vi "Multi-output Decision Tree Regression.vi"() -> ()   [LabVIEW 2020]
doc: "An example to illustrate multi-output regression with decision tree.\n\nThe decision trees is used to predict simultaneously the noisy x and y observations of a circle given a single underlying feature. As a result, it learns local linear regressions approximating the circle.\n\nWe can see that if the maximum depth of the tree (controlled by the max_depth parameter) is set too high, the decision trees learn too fine details of the training data and learn from the noise, i.e. they overfit."
uses:
  Model/Supervised/Tree/DecisionTreeRegressor/Controls/decision_tree_regressor_params.ctl
  Model/Supervised/Tree/DecisionTreeRegressor/DecisionTreeRegressor.lvclass
  C:/Users/cipop/TDF Dropbox/2_Technologies de France/1 - Services et Etudes/PLAIY/2 - DEV/PLAIYLAB/code/Model/Model.lvclass
  C:/Users/cipop/TDF Dropbox/2_Technologies de France/1 - Services et Etudes/PLAIY/2 - DEV/PLAIYLAB/code/Model/Supervised/Tree/Tree.lvclass
  Model/Supervised/Tree/DecisionTreeRegressor/DecisionTreeRegressor.vi
panel:
  in  "error in":errorcluster
  in  "X_test":dbl[][](array[numeric])=array20000x1[20000 elements]
  in  "Y":dbl[][](array[numeric])=[[1.8256976133184155, 2.6449015931558], [2.8069433208733265, 1.4109123270047574], [-2.720432252800947, -1.5712583361782755], [-2.993723955966916, -0.9524816410614725], [-0.852188059374447, 3.0238022277505143], [2.3890282910556984, -1.3300710818645851], [-2.7953490289874754, -1.4337462143727313], [-3.0739434689186576, 0.6484411700236866], [-3.035155908655832, 0.8108224289207518], [0.4667646891222363, 3.106724179272756], [2.657323005508145, 0.5622915200653608], [2.6321235585609952, -1.7150889112689056], [2.2861793518787192, -2.1547594696700503], [-3.131091686155956, -0.25665006131775714], [3.09796044300452, 0.52177149660421], [1.2566356253877626, -3.4745833366109107], [-0.3508125342066263, -3.1219441005458255], [-1.029946994677885, -2.967964553232291], [-3.1400292397187446, 0.09909982240488503], [-3.139440982914441, 0.11625281023083907], [2.374924854338179, -2.310100563289901], [0.1898574871704973, -3.135850528270546], [0.26325593502023165, 3.1305431978757268], [1.998387653083125, -2.424056762762431], [-1.7235342528252657, -2.6266012412293214], [-2.507857486775842, 1.715435086269062], [-2.2807611493251936, -2.1604936891410214], [-0.7260634523667222, -3.0565399170020133], [-2.813177057014104, -1.3984417209804716], [0.22316518691925616, 3.1336562830720043], [2.7072417339618564, -0.09180969787531168], [1.328074566794052, -2.8470725923523883], [-3.0330950538704733, -0.8184978895976633], [1.1767886156655354, 2.9128633601886222], [2.258533538271828, 2.1837194548729686], [2.0169505446781475, 2.4581823603746082], [2.5898528068960425, 1.778276367638632], [2.9230441084338596, 1.1512677973605707], [-3.061595888228995, -0.704439506465011], [-3.138513218222494, -0.13906538078199607], [1.1882465114137004, 2.3680122824827508], [3.128889883239954, -0.2822277442917763], [3.1209808517306605, -0.35928112143545593], [2.4365611927984574, -1.9831222743033061], [2.320560298326097, -2.117688433864163], [1.163818201165327, -2.4488127202110106], [0.22133561986844763, -3.1337860399948823], [-3.0480845941241945, -0.7607790140061058], [2.6376306285752116, -1.7066074734077816], [1.7551500436024252, -2.6055810725309936], [-2.640875958769442, 0.11463798380303492], [0.5122025995369903, -3.099556887381954], [1.0768665573344194, 2.9512646134808165], [2.4532511789429097, 1.96243803828416], [3.1286979062077664, 0.2843480486665858], [-1.8432014614152683, 2.377668793227683], [2.595118339887417, -1.7705832945866549], [2.430215435157508, -1.9908936033378486], [0.09436047647264918, -3.1401752342137232], [-3.1399592202002538, 0.10129410925011163], [-2.9838035181445264, 1.6890017291269777], [-3.1138635263815986, -0.4164833011775086], [-2.2395802491581875, 2.20315335568587], [-1.2184723923859657, 2.8956742617363886], [3.002738180455847, 0.923670840030184], [3.0076138641555845, 0.3674314765799399], [1.4060012437714013, -2.8094065038015823], [-2.9388665139979615, -1.1102558326758865], [-1.9142577560461527, 2.4910282303712465], [-1.2202862616970438, 2.894910333775955], [2.3422131280375744, 2.6709038209071414], [2.1766010669755884, 2.265394490222418], [2.9058348451257574, 1.1940386316791947], [2.4393286440630204, -1.9797171937787035], [0.25920539036144385, 3.13088118054597], [2.8615826236106736, 0.6179612178483794], [-1.8568171941699843, 2.5341338379264946], [-0.7364447224204342, 3.054055266675514], [-0.3232054114594505, 3.124922825141876], [-0.24165004579056773, 3.1322850535126547], [2.972047565800148, 1.299914590322177], [-1.3909118919367747, -2.8169076147360994], [-3.0677792098733216, 0.6770045203382145], [-2.5585023948376673, -1.8230934964228462], [-0.37731343682908297, 3.1188521881419105], [0.4010838370305029, 3.32924687119214], [0.717059789905144, 3.0586646855761335], [2.9939436325287945, 0.9517909047315192], [-1.1697036424392835, -2.915715656567634], [-1.8696557692167248, -2.524676554674673], [-2.959968196291449, 1.7949709876659181], [-2.64529910590806, 1.6946967402374318], [0.1183836979789325, 3.1393613524317634], [-1.972269507042122, -2.4453542468691896], [2.5633577388920226, 1.8162603072114238], [2.5739321091870977, -1.3610566109470112], [-1.4275971586239513, -2.7984943726543707], [-3.009488498821716, 0.9014340666677573], [-1.762098393366606, 2.6008870896646368], [-1.173578057741207, -2.914158359368573]]
  in  "X":dbl[][](array[numeric])=[[-99.97712503653102], [-99.4259345937682], [-96.34234453116164], [-96.12660842594059], [-94.52248136041477], [-92.18904335342353], [-90.00930821078256], [-89.32749097658393], [-82.99115772604442], [-81.53228104624044], [-80.33063323338999], [-79.53311423443483], [-79.3547986844716], [-77.05080540932497], [-73.99428557634447], [-72.5050591707525], [-72.14473054984829], [-71.92261228095325], [-70.65428501883797], [-70.64882183657738], [-66.92916057661344], [-66.03391608708623], [-62.74795772446582], [-60.37970218302424], [-59.109550053696516], [-57.674376799988195], [-52.59460395139446], [-46.890668125554754], [-46.01442164699478], [-43.91120158711897], [-42.44493228273025], [-41.2771703252641], [-39.53348547363205], [-37.31516436815143], [-36.89687379878741], [-30.88785459139045], [-30.446828050898688], [-30.220331604431493], [-20.646505153866016], [-20.46463260289329], [-18.372639447743765], [-17.188802436086334], [-17.16414609461947], [-16.595599059485195], [-16.539039526574612], [-16.161097119341036], [-15.778474998989566], [-14.381762025741011], [-10.421294764818967], [-10.01757330401189], [-1.6853681439323367], [2.9778224116617196], [6.6330569946034075], [7.179281183102319], [7.7633468006713855], [11.737965689150329], [14.735897334457178], [14.823521098402608], [15.677922877426354], [17.31100810039858], [17.861107380656847], [23.428982724144774], [24.339144041824355], [24.73444141112178], [32.68829956368961], [32.75892904395775], [34.093502035680444], [35.76710658797819], [37.043900079351886], [37.30018553631675], [38.37542279009466], [38.464523133862826], [38.88003154554903], [39.951672004186236], [44.06489868843161], [45.199597070090306], [49.63313087596788], [50.028862988993495], [50.162420627231114], [50.18848680546745], [57.85586569029769], [60.14891373510733], [61.47825774190477], [66.92513437947457], [75.27783045920765], [75.62348727818909], [75.62850068588261], [76.66121824116198], [78.92133270076945], [79.17724363921337], [80.67590411245075], [80.6803830575767], [81.71910061861911], [85.50171607920677], [88.91895119816266], [89.89785174141426], [91.5779060301004], [92.96800942967712], [93.65231514387949], [97.77221778129893]]
  out "error out":errorcluster caption="sortie d'erreur"
  out "XY Graph":cluster{"X":dbl[], "Y":dbl[]}[](graph) caption="Multi-outpout Decision Tree Regression"
  out "y_3":dbl[][](array[numeric])
  out "y_2":dbl[][](array[numeric])
  out "y_1":dbl[][](array[numeric])
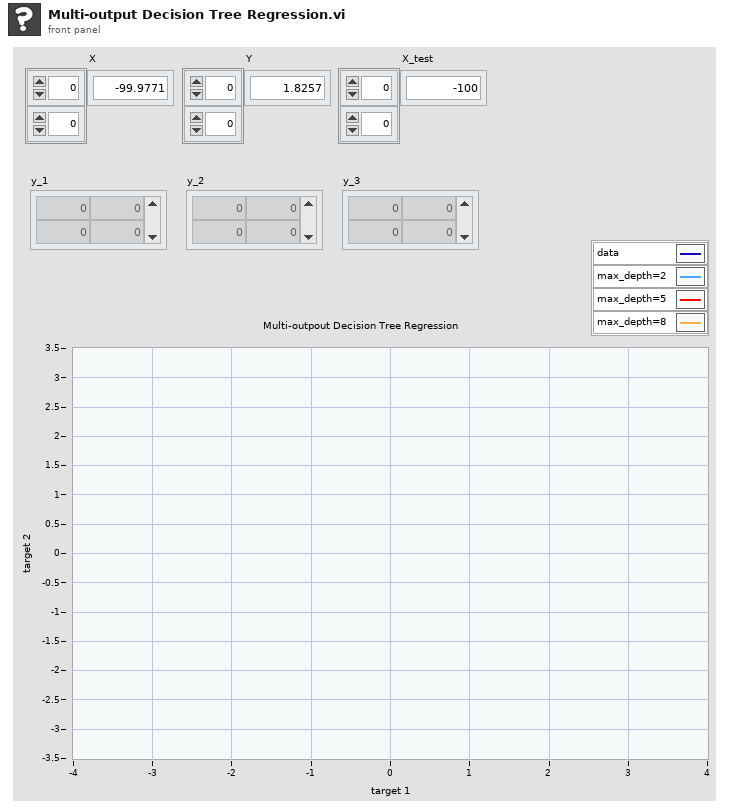
[diagram p1: front panel]
types:
  T1 = cluster{"max_depth_type":string, "max_depth_int":dbl}
  T2 = typedef "decision_tree_regressor_params.ctl" = cluster{"criterion":string, "splitter":string, "max_depth":cluster{"max_depth_type":string, "max_depth_int":dbl}, "min_samples_split":dbl, "min_samples_leaf":dbl, "min_weight_fraction_leaf":dbl, "max_features":cluster{"max_features_type":string, "max_features_int":dbl, "max_features_float":dbl}, "random_state":dbl, "max_leaf_nodes":cluster{"max_leaf_nodes_type":string, "max_leaf_nodes_int":dbl}, "min_impurity_decrease":dbl, "ccp_alpha":dbl}
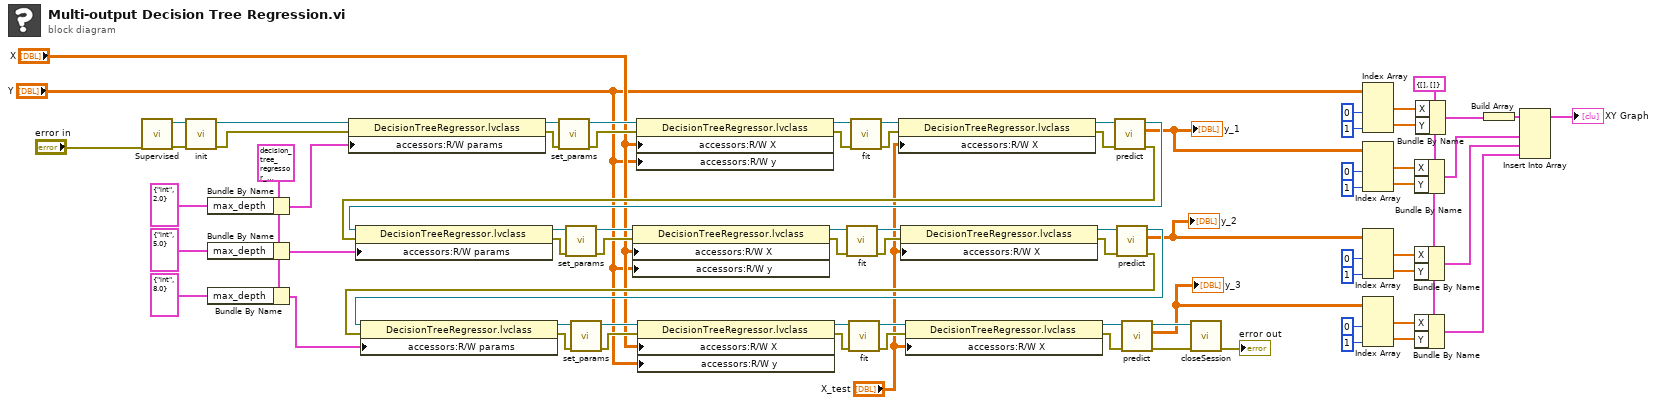
[diagram p0: block diagram]
diagram:
  w7 = cluster{"X":dbl[], "Y":dbl[]} {"X"=[], "Y"=[]}
  w44 = T2 {"criterion"="mse", "splitter"="best", "max_depth"={"max_depth_type"="None", "max_depth_int"=0.0}, "min_samples_split"=2.0, "min_samples_leaf"=1.0, "min_weight_fraction_leaf"=0.0, "max_features"={"max_features_type"="None", "max_features_int"=0.0, "max_features_float"=0.0}, "random_state"=0.0, "max_leaf_nodes"={"max_leaf_nodes_type"="None", "max_leaf_nodes_int"=0.0}, "min_impurity_decrease"=0.0, "ccp_alpha"=0.0} ("R/W params")
  n1 = call-poly "Supervised.vi"("error in"="error in") -> ("error out"=w76:errorcluster, "out"=w77:refnum<class "DecisionTreeRegressor.lvclass">)  [unwired: 9 in]
  n2 = call-dynamic "init.vi"("error in (no error)"=w76, "Model en entrée"=w77) -> ("error out"=w74:errorcluster, "Model en sortie"=w75:refnum<class "DecisionTreeRegressor.lvclass">)  [unwired: 8 in]
  n3 = Bundle By Name(cluster=w44, "max_depth"=T1 {"max_depth_type"="int", "max_depth_int"=2.0}) -> (w49:T2)
  n4 = Bundle By Name(cluster=w44, "max_depth"=T1 {"max_depth_type"="int", "max_depth_int"=5.0}) -> (w47:T2)
  n5 = Bundle By Name(cluster=w44, "max_depth"=T1 {"max_depth_type"="int", "max_depth_int"=8.0}) -> (w45:T2)
  n6 = property class="DecisionTreeRegressor.lvclass"(reference=w75, error in=w74, "accessors:R/W params"=w49) -> (reference out=w73:refnum<class "DecisionTreeRegressor.lvclass">, error out=w72:errorcluster)
  n7 = call-dynamic "set_params.vi"("error in (no error)"=w72, "DecisionTreeRegressor.lvclass 2"=w73) -> ("error out"=w78:errorcluster, "DecisionTreeRegressor.lvclass"=w71:refnum<class "DecisionTreeRegressor.lvclass">)  [unwired: 8 in]
  n8 = property class="DecisionTreeRegressor.lvclass"(reference=w71, error in=w78, "accessors:R/W X"="X", "accessors:R/W y"="Y") -> (reference out=w70:refnum<class "DecisionTreeRegressor.lvclass">, error out=w69:errorcluster)
  n9 = call-dynamic "fit.vi"("error in (no error)"=w69, "Tree.lvclass 2"=w70) -> ("error out"=w5:errorcluster, "Tree.lvclass"=w68:refnum<class "DecisionTreeRegressor.lvclass">)  [unwired: 8 in]
  n10 = property class="DecisionTreeRegressor.lvclass"(reference=w68, error in=w5, "accessors:R/W X"="X_test") -> (reference out=w67:refnum<class "DecisionTreeRegressor.lvclass">, error out=w66:errorcluster)
  n11 = call-dynamic "predict.vi"("error in (no error)"=w66, "Tree.lvclass 2"=w67) -> ("error out"=w43:errorcluster, "C"=w24:dbl[][], "Tree.lvclass"=w42:refnum<class "DecisionTreeRegressor.lvclass">)  [unwired: 7 in]
  "y_1" <- w24
  n12 = property class="DecisionTreeRegressor.lvclass"(reference=w42, error in=w43, "accessors:R/W params"=w47) -> (reference out=w62:refnum<class "DecisionTreeRegressor.lvclass">, error out=w63:errorcluster)
  n13 = call-dynamic "set_params.vi"("error in (no error)"=w63, "DecisionTreeRegressor.lvclass 2"=w62) -> ("error out"=w39:errorcluster, "DecisionTreeRegressor.lvclass"=w61:refnum<class "DecisionTreeRegressor.lvclass">)  [unwired: 8 in]
  n14 = property class="DecisionTreeRegressor.lvclass"(reference=w61, error in=w39, "accessors:R/W X"="X", "accessors:R/W y"="Y") -> (reference out=w40:refnum<class "DecisionTreeRegressor.lvclass">, error out=w64:errorcluster)
  n15 = call-dynamic "fit.vi"("error in (no error)"=w64, "Tree.lvclass 2"=w40) -> ("error out"=w37:errorcluster, "Tree.lvclass"=w38:refnum<class "DecisionTreeRegressor.lvclass">)  [unwired: 8 in]
  n16 = property class="DecisionTreeRegressor.lvclass"(reference=w38, error in=w37, "accessors:R/W X"="X_test") -> (reference out=w36:refnum<class "DecisionTreeRegressor.lvclass">, error out=w65:errorcluster)
  n17 = call-dynamic "predict.vi"("error in (no error)"=w65, "Tree.lvclass 2"=w36) -> ("error out"=w41:errorcluster, "C"=w14:dbl[][], "Tree.lvclass"=w35:refnum<class "DecisionTreeRegressor.lvclass">)  [unwired: 7 in]
  "y_2" <- w14
  n18 = property class="DecisionTreeRegressor.lvclass"(reference=w35, error in=w41, "accessors:R/W params"=w45) -> (reference out=w52:refnum<class "DecisionTreeRegressor.lvclass">, error out=w53:errorcluster)
  n19 = call-dynamic "set_params.vi"("error in (no error)"=w53, "DecisionTreeRegressor.lvclass 2"=w52) -> ("error out"=w51:errorcluster, "DecisionTreeRegressor.lvclass"=w54:refnum<class "DecisionTreeRegressor.lvclass">)  [unwired: 8 in]
  n20 = property class="DecisionTreeRegressor.lvclass"(reference=w54, error in=w51, "accessors:R/W X"="X", "accessors:R/W y"="Y") -> (reference out=w55:refnum<class "DecisionTreeRegressor.lvclass">, error out=w56:errorcluster)
  n21 = call-dynamic "fit.vi"("error in (no error)"=w56, "Tree.lvclass 2"=w55) -> ("error out"=w58:errorcluster, "Tree.lvclass"=w57:refnum<class "DecisionTreeRegressor.lvclass">)  [unwired: 8 in]
  n22 = property class="DecisionTreeRegressor.lvclass"(reference=w57, error in=w58, "accessors:R/W X"="X_test") -> (reference out=w59:refnum<class "DecisionTreeRegressor.lvclass">, error out=w60:errorcluster)
  n23 = call-dynamic "predict.vi"("error in (no error)"=w60, "Tree.lvclass 2"=w59) -> ("error out"=w33:errorcluster, "C"=w9:dbl[][], "Tree.lvclass"=w34:refnum<class "DecisionTreeRegressor.lvclass">)  [unwired: 7 in]
  "y_3" <- w9
  n24 = call-dynamic "closeSession.vi"("error in"=w33, "Python en entrée"=w34) -> ("error out"=→"error out":errorcluster)  [unwired: 8 in, 1 out]
  n25 = Index Array(array="Y", index (col) #1=0 ("disabled index (col)"), index (col) #2=1 ("index (col)")) -> (element #1=w28:dbl[], element #2=w27:dbl[])  [unwired: 2 in]
  n26 = Index Array(array=w24, index (col) #1=0 ("disabled index (col)"), index (col) #2=1 ("index (col)")) -> (element #1=w23:dbl[], element #2=w22:dbl[])  [unwired: 2 in]
  n27 = Index Array(array=w14, index (col) #1=0 ("disabled index (col)"), index (col) #2=1 ("index (col)")) -> (element #1=w17:dbl[], element #2=w18:dbl[])  [unwired: 2 in]
  n28 = Index Array(array=w9, index (col) #1=0 ("disabled index (col)"), index (col) #2=1 ("index (col)")) -> (element #1=w8:dbl[], element #2=w10:dbl[])  [unwired: 2 in]
  n29 = Bundle By Name(cluster=w7, "X"=w23, "Y"=w22) -> (w20:cluster{"X":dbl[], "Y":dbl[]})
  n30 = Bundle By Name(cluster=w7, "X"=w17, "Y"=w18) -> (w13:cluster{"X":dbl[], "Y":dbl[]})
  n31 = Bundle By Name(cluster=w7, "X"=w8, "Y"=w10) -> (w6:cluster{"X":dbl[], "Y":dbl[]})
  n32 = Bundle By Name(cluster=w7, "X"=w28, "Y"=w27) -> (w31:cluster{"X":dbl[], "Y":dbl[]})
  n33 = Build Array(w31) -> (w21:cluster{"X":dbl[], "Y":dbl[]}[])
  n34 = Insert Into Array(array=w21, new element #1=w20, new element #2=w13, new element #3=w6) -> (→"XY Graph":cluster{"X":dbl[], "Y":dbl[]}[])  [unwired: 1 in]
